vi "WS1021 I2C Monitor Single Board.vi"(5 "SN Brd B":string[](array[string]), 7 "SN Brd A":string[](array[string]), 8 "Error In":errorcluster, 11 "AD7747 Values":string[][](table)) -> (0 "Error Out":errorcluster, 1 "I2C Board B":string[][](table), 3 "I2C Board A":string[][](table))   [LabVIEW 2017]
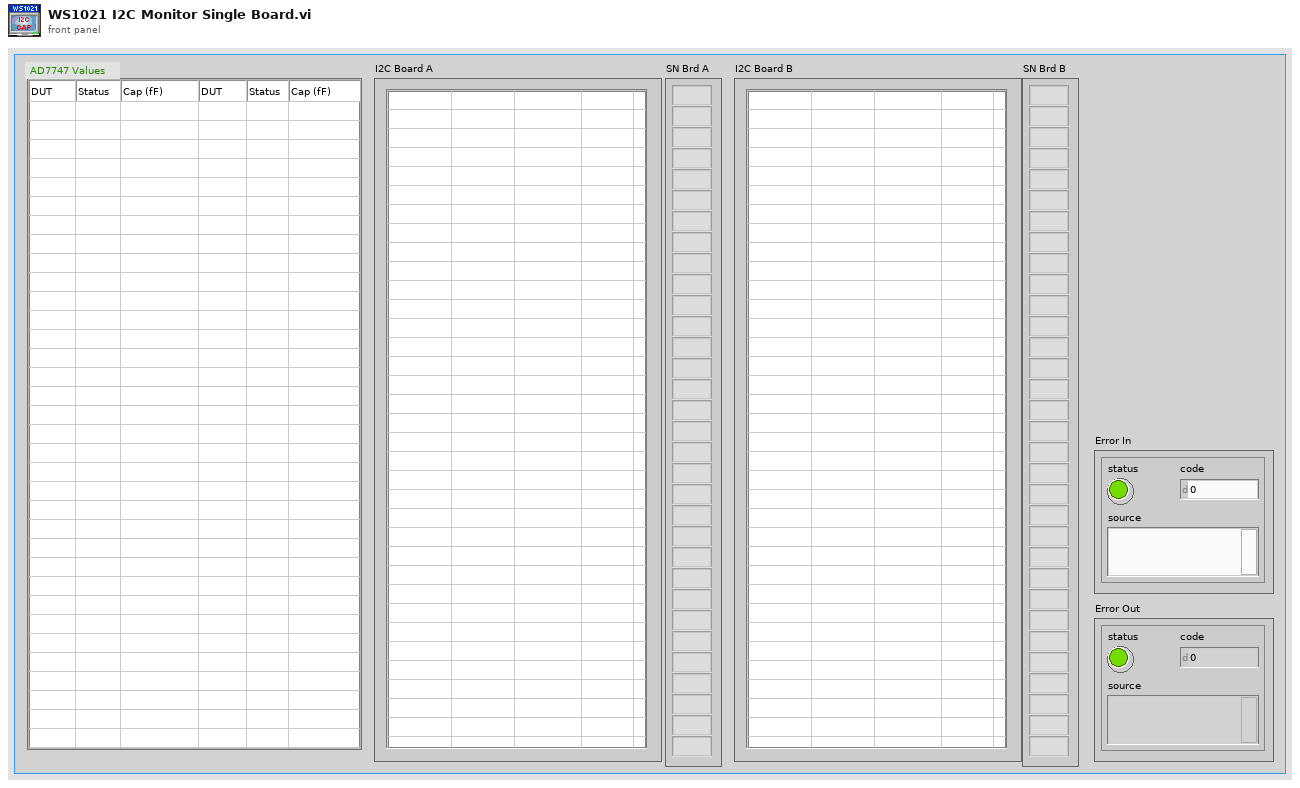
[diagram p1: front panel]
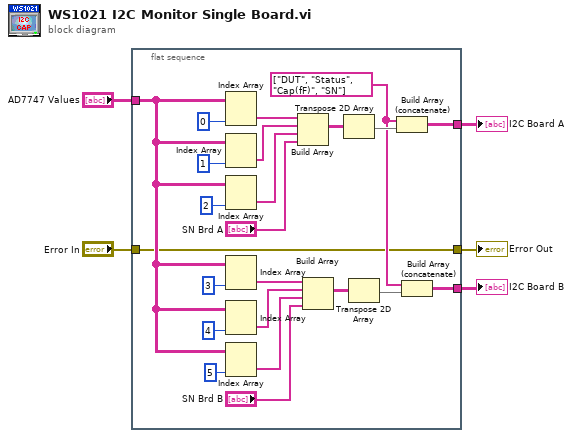
[diagram p0: block diagram]
diagram:
  n1 = flat-sequence {
    tunnel: [w21] -> w5
    tunnel: "AD7747 Values" -> [w11]
    tunnel: [w10] -> w3
    tunnel: "Error In" -> [w6]
    tunnel: [w6] -> w1
    frame #0 {
      w9 = string[] ["DUT", "Status", "Cap(fF)", "SN"] ("element")
      n2 = Index Array(array=w11, index (col)=0 ("disabled index (col)")) -> (element=w25:string[])  [unwired: 1 in]
      n3 = Index Array(array=w11, index (col)=1 ("disabled index (col)")) -> (element=w24:string[])  [unwired: 1 in]
      n4 = Index Array(array=w11, index (col)=2 ("disabled index (col)")) -> (element=w23:string[])  [unwired: 1 in]
      n5 = Index Array(array=w11, index (col)=3 ("disabled index (col)")) -> (element=w15:string[])  [unwired: 1 in]
      n6 = Index Array(array=w11, index (col)=4 ("disabled index (col)")) -> (element=w16:string[])  [unwired: 1 in]
      n7 = Index Array(array=w11, index (col)=5 ("disabled index (col)")) -> (element=w17:string[])  [unwired: 1 in]
      n8 = Build Array(w25, w24, w23, "SN Brd A") -> (w22:string[][])
      n9 = Build Array(w15, w16, w17, "SN Brd B") -> (w18:string[][])
      n10 = Transpose 2D Array(2D array=w22) -> (transposed array=w20:string[][])
      n11 = Transpose 2D Array(2D array=w18) -> (transposed array=w19:string[][])
      n12 = Build Array (concatenate)(w9, w20) -> (w21:string[][])
      n13 = Build Array (concatenate)(w9, w19) -> (w10:string[][])
    }
  }
  "I2C Board A" <- w5
  "I2C Board B" <- w3
  "Error Out" <- w1
